vi "List Package BuildSpec MinVersion Dependencies.vi"(8 "error in (no error)":errorcluster, 10 "package buildspec ref in":refnum<vi>, 11 "project ref in":refnum<vi>) -> (0 "error out":errorcluster, 2 "package buildspec ref out":refnum<vi>, 3 "project ref out":refnum<vi>, 4 "dependency package names":string[](array[string]), 6 "dependency package min versions":string[](array[string]))   [LabVIEW 2018, in "NIPKG BuildSpec API.lvlib"]
uses:
  NIPKG BuildSpec API.lvlib
panel:
  out "# of dependencies":i32
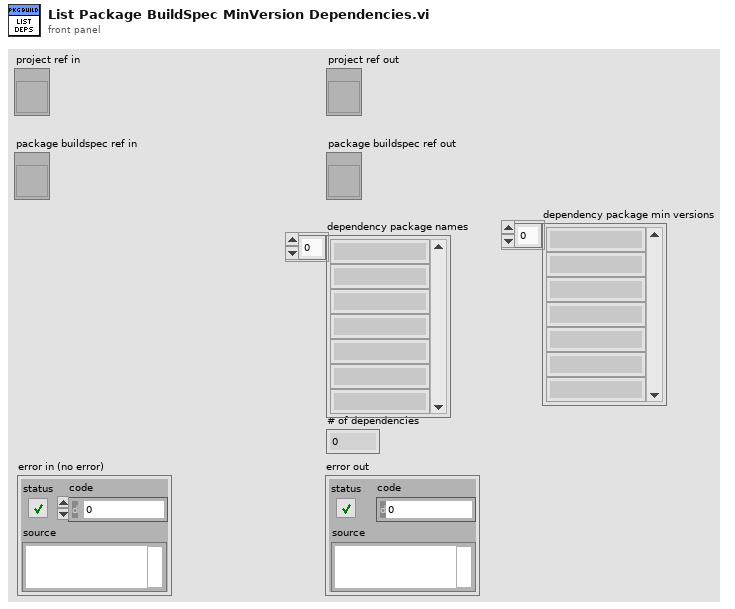
[diagram p1: front panel]
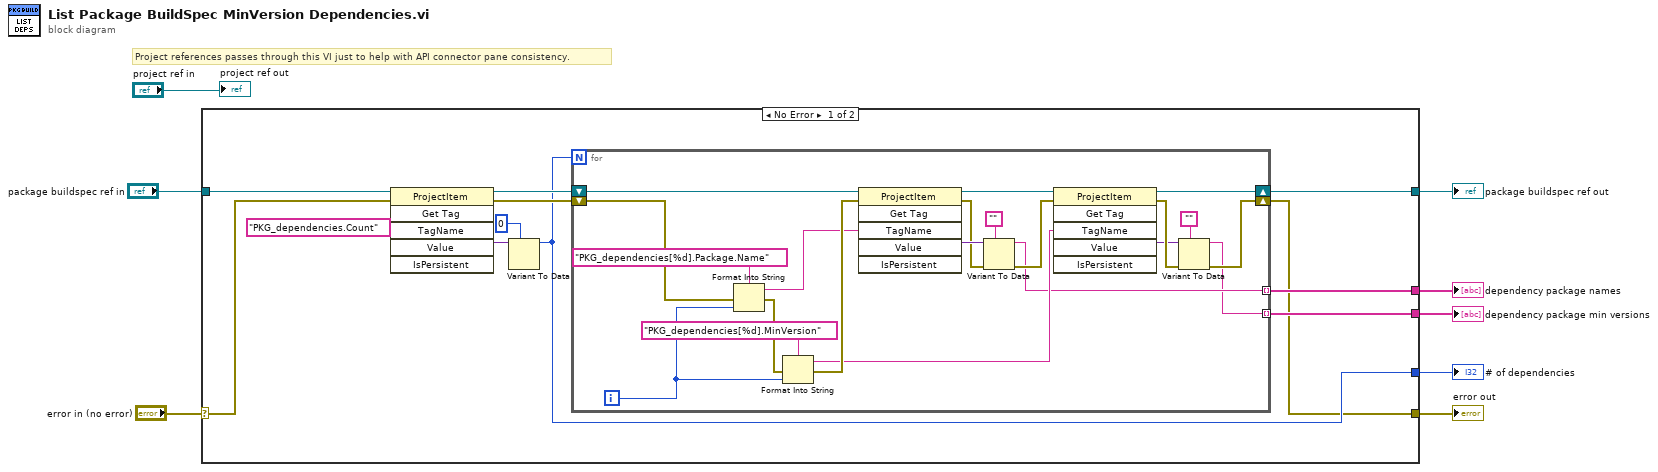
[diagram p0: block diagram]
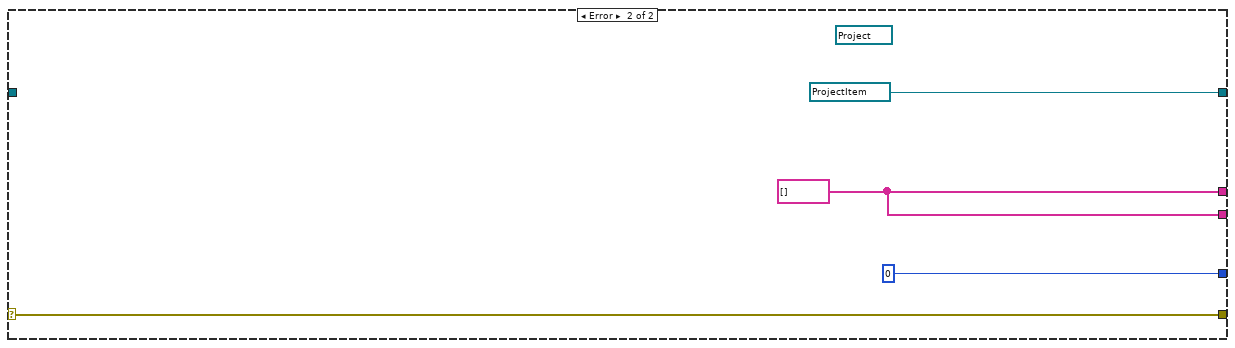
[diagram p2: hidden frame]
diagram:
  # "Project references passes through this VI just to help with API connector pane consistency."
  n1 = case shown="No Error" "error in (no error)" {
    selector: "error in (no error)" -> [w15 w45]
    tunnel: "package buildspec ref in" -> [w16 _]
    tunnel: [w9 w45] -> w2
    tunnel: [w13 refnum<vi> refnum ("package buildspec ref in")] -> w7
    tunnel: [w12 0] -> w5
    tunnel: [w11 w42] -> w3
    tunnel: [w10 w42] -> w4
    frame No Error {
      n2 = invoke class="ProjectItem" method="Get Tag"(reference=w16, error in=w15, "TagName"="PKG_dependencies.Count" ("Tag Name")) -> (reference out=w17:refnum<vi>, error out=w14:errorcluster, "Value"=w19:variant)  [unwired: 3 in, 3 out]
      n3 = Variant To Data(type=0, Variant=w19) -> (data=w12:i32)  [unwired: 1 in, 1 out]
      n4 = for {
        N: w12 -> [_]
        shift-right: [w25] -> w9
        shift-left: w14 -> [w37]
        shift-right: [w27] -> w13
        shift-left: w17 -> [w39]
        tunnel: [w22] -> w10 mode=indexing
        tunnel: [w21] -> w11 mode=indexing
        i -> [w35]
        n5 = Format Into String(format string="PKG_dependencies[%d].Package.Name", error in=w37, w35) -> (resulting string=w23:string, error out=w33:errorcluster)  [unwired: 1 in]
        n6 = Format Into String(format string="PKG_dependencies[%d].MinVersion", error in=w33, w35) -> (resulting string=w24:string, error out=w32:errorcluster)  [unwired: 1 in]
        n7 = invoke class="ProjectItem" method="Get Tag"(reference=w39, error in=w32, "TagName"=w23) -> (reference out=w28:refnum<vi>, error out=w36:errorcluster, "Value"=w41:variant)  [unwired: 3 in, 3 out]
        n8 = Variant To Data(error in=w36, type="", Variant=w41) -> (data=w22:string, error out=w26:errorcluster)
        n9 = invoke class="ProjectItem" method="Get Tag"(reference=w28, error in=w26, "TagName"=w24) -> (reference out=w27:refnum<vi>, error out=w31:errorcluster, "Value"=w29:variant)  [unwired: 3 in, 3 out]
        n10 = Variant To Data(error in=w31, type="", Variant=w29) -> (data=w21:string, error out=w25:errorcluster)
      }
    }
    frame Error {
      w42 = string[] []
      (unwired) refnum<vi> refnum ("project ref in")
    }
  }
  "package buildspec ref out" <- w7
  "# of dependencies" <- w5
  "dependency package names" <- w4
  "dependency package min versions" <- w3
  "error out" <- w2
  "project ref out" <- "project ref in"
